vi "FGV_READ.vi"(7 "States":T2=enum."Close Comm", 8 "error in":errorcluster, 11 "Item":T1(array[cluster])=[{"Item"=enum."Urms", "Ch(0:Ch1)"=enum."1"}, {"Item"=enum."Urms", "Ch(0:Ch1)"=enum."2"}, {"Item"=enum."Urms", "Ch(0:Ch1)"=enum."3"}, {"Item"=enum."Urms", "Ch(0:Ch1)"=enum."4"}]) -> (0 "error out":errorcluster, 3 "Data out":dbl[](array[numeric]))   [LabVIEW 2018]
uses:
  Conotrls/States.ctl
  PW3390/Common/_Initialize/HIOKI PW3390 Initialize LAN.vi
panel:
  out "4th data 2":dbl(graph)
  out "3rd data 2":dbl(graph)
  out "2nd data 2":dbl(graph)
  out "1st data 2":dbl(graph)
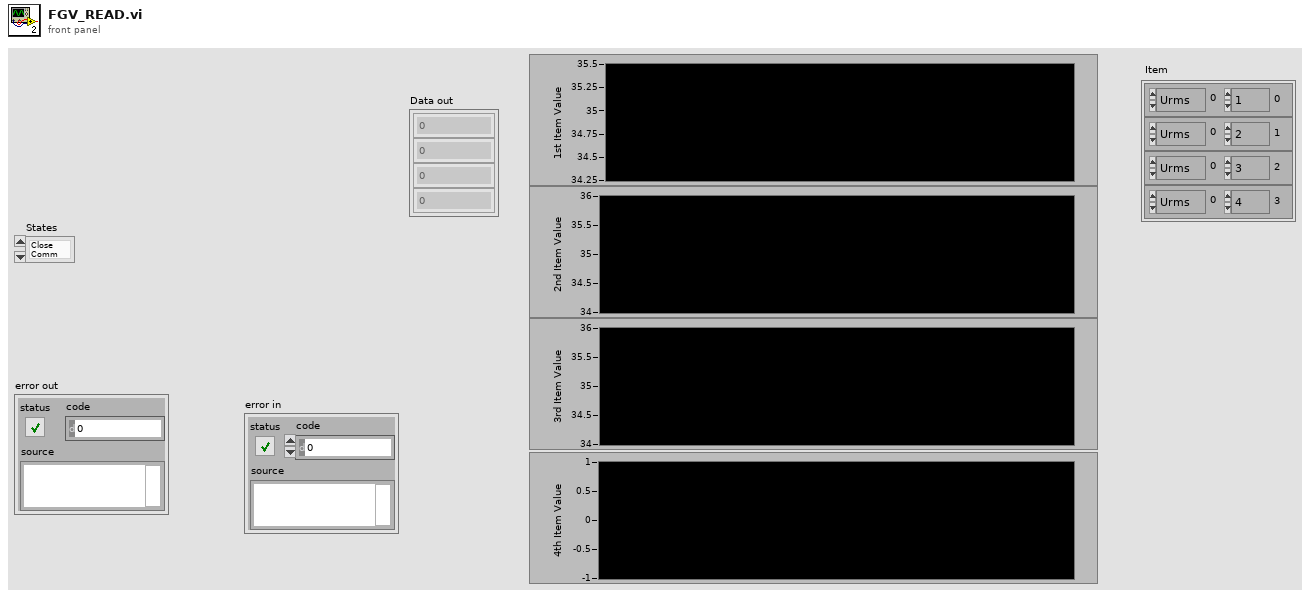
[diagram p1: front panel]
types:
  T1 = cluster{"Item":enum16{"Urms", "Umn", "Uac", "Udc", "Ufnd", "Upk+", "Upk-", "Uthd", "Urf", "Uunb", "Irms", "Imn", "Iac", "Idc", "Ifnd", "Ipk+", "Ipk-", "Ithd", "Irf", "Iunb", "P", "S", "Q", "PF", "DEG U", "DEG I", "DEG P", "f", "EFFI", "LOSS", "IH+", "IH-", "IH", "WP+", "WP-", "WP", "CH A", "CH B", "Pm", "Slip", "Laptime", "Laptime(ms)"}, "Ch(0:Ch1)":enum16{"1", "2", "3", "4", "12", "34", "123"}}[]
  T2 = typedef "States.ctl" = enum16{"Open Com", "Read Data", "Close Comm"}
  T3 = cluster{"VISA Resource out":refnum<visa-resource-name>}
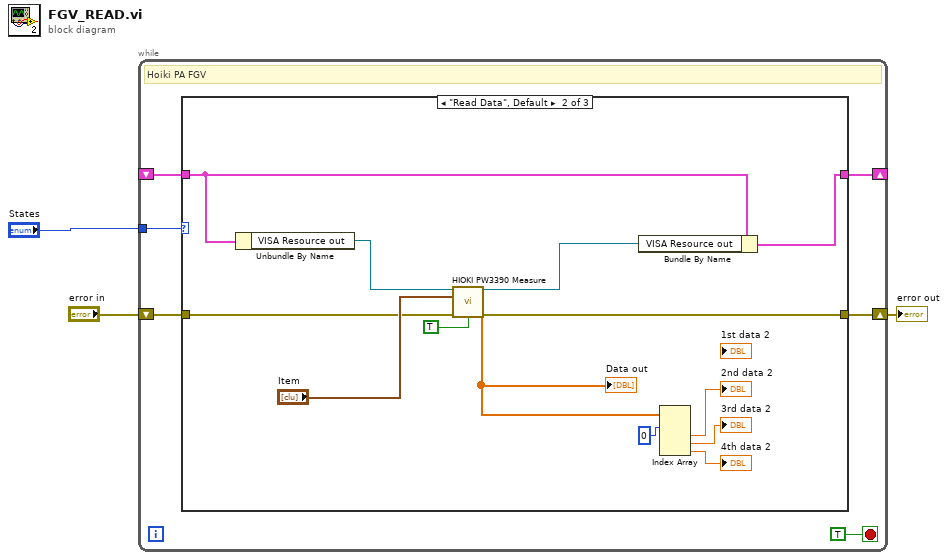
[diagram p0: block diagram]
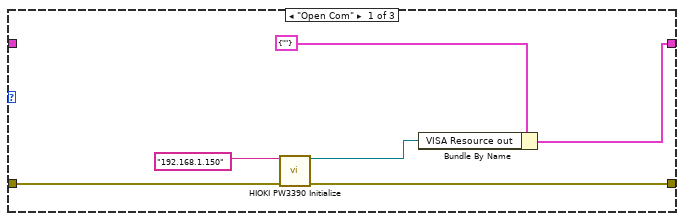
[diagram p2: hidden frame]
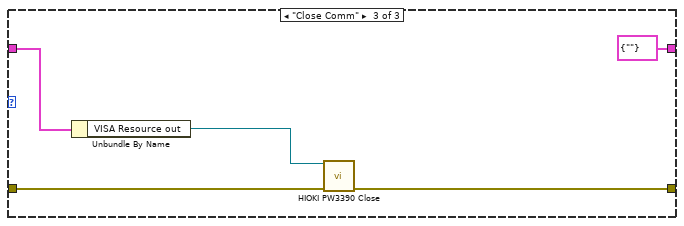
[diagram p3: hidden frame]
diagram:
  n1 = while {
    tunnel: "States" -> [w8]
    shift-right: [w7] -> _
    shift-left: _ -> [w4]
    shift-right: [w6] -> w1
    shift-left: "error in" -> [w5]
    stop <- TRUE stop-if-true
    # "Hoiki PA FGV"
    n2 = case shown="\"Read Data\", Default" w8 {
      tunnel: [w13 w17 T3 {"VISA Resource out"=""}] -> w7
      tunnel: [w11 w20 w32] -> w6
      tunnel: w5 -> [w10 w21 w33]
      tunnel: w4 -> [_ w18 w31]
      frame "Open Com" {
        n3 = call-poly "HIOKI PW3390 Initialize.vi"("IP Address"="192.168.1.150" ("IP Address 2"), "error in (no error)"=w10) -> ("VISA Resource out"=w12:refnum<visa-resource-name>, "error out"=w11:errorcluster)  [unwired: 11 in, 1 out]
        n4 = Bundle By Name(cluster=T3 {"VISA Resource out"=""}, "VISA Resource out"=w12) -> (w13:T3)
      }
      frame "Read Data", Default {
        n5 = Unbundle By Name(w18) -> ("VISA Resource out"=w19:refnum<visa-resource-name>)
        n6 = call "HIOKI PW3390 Measure.vi"("VISA Resource"=w19, "Item"="Item", "error in (no error)"=w21, "Error Out (F: Off)"=TRUE) -> ("VISA Resource out"=w16:refnum<visa-resource-name>, "Data out"=w28:dbl[], "error out"=w20:errorcluster)  [unwired: 6 in, 3 out]
        "Data out" <- w28
        n7 = Bundle By Name(cluster=w18, "VISA Resource out"=w16) -> (w17:T3)
        n8 = Index Array(array=w28, index #1=0 ("Žw•W")) -> (element #2=→"2nd data 2":dbl, element #3=→"3rd data 2":dbl, element #4=→"4th data 2":dbl)  [unwired: 3 in, 1 out]
      }
      frame "Close Comm" {
        n9 = Unbundle By Name(w31) -> ("VISA Resource out"=w30:refnum<visa-resource-name>)
        n10 = call "HIOKI PW3390 Close.vi"("VISA Resource"=w30, "error in (no error)"=w33) -> ("error out"=w32:errorcluster)  [unwired: 13 in]
      }
    }
  }
  "error out" <- w1
